vi "New.vi"(8 "error in (no error)":errorcluster) -> (0 "error out":errorcluster, 3 "BlueTOMLSerializer out":refnum<class "BlueTOMLSerializer.lvclass">)   [LabVIEW 2019, in "BlueTOMLSerializer.lvlib" / "BlueTOMLSerializer.lvclass"]
uses:
  BlueTOMLSerializer.lvclass
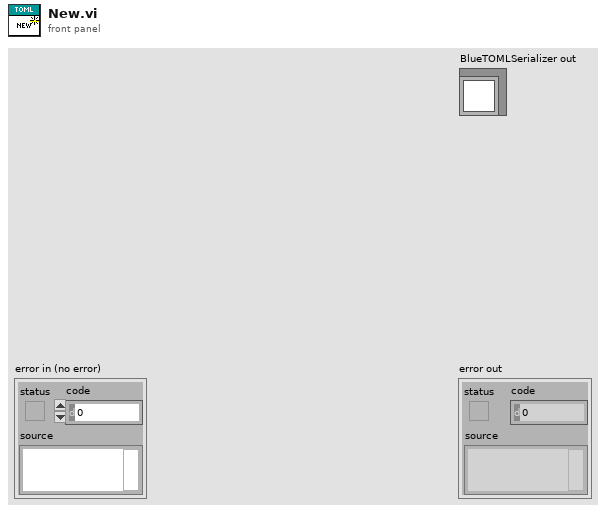
[diagram p1: front panel]
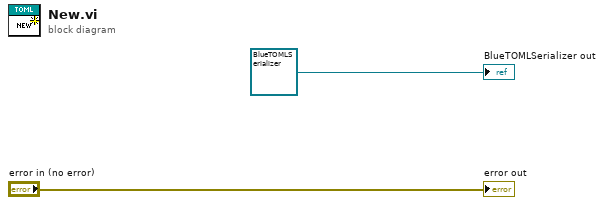
[diagram p0: block diagram]
diagram:
  "error out" <- "error in (no error)"
  "BlueTOMLSerializer out" <- refnum<class "BlueTOMLSerializer.lvclass"> refnum ("BlueTOMLSerializer out")
